vi "getFilePath.vi"(11 "fileName":string="VI\\SYSKON P4500 Init Config.vi") -> (3 "path":path=path "C:/Users/chen106/Desktop/vTestStudioCfgEditor/VI/SYSKON P4500 Init Config.vi")   [LabVIEW 2010]
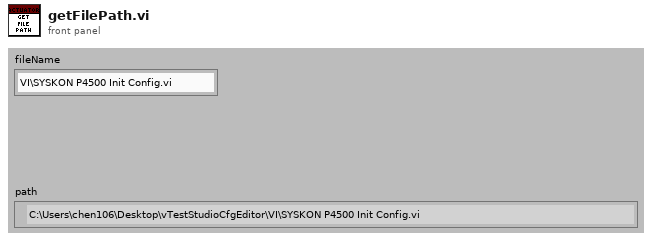
[diagram p1: front panel]
types:
  T1 = enum32{"invalid app kind", "Development System", "Run Time System", "Student Edition", "Embedded LabVIEW", "Evaluation", "Custom"}
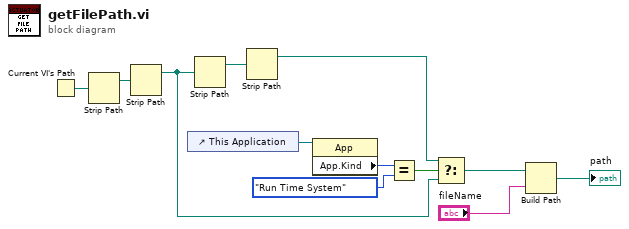
[diagram p0: block diagram]
diagram:
  n1 = Current VI's Path() -> (path=w12:path)
  n2 = Strip Path(path=w12) -> (stripped path=w10:path)  [unwired: 1 out]
  n3 = Strip Path(path=w10) -> (stripped path=w3:path)  [unwired: 1 out]
  n4 = control-ref of="This Application"() -> (w9:refnum<vi>)
  n5 = Strip Path(path=w3) -> (stripped path=w5:path)  [unwired: 1 out]
  n6 = Strip Path(path=w5) -> (stripped path=w4:path)  [unwired: 1 out]
  n7 = property class="App"(reference=w9) -> ("App.Kind"=w8:T1)  [unwired: 1 in, 2 out]
  n8 = Equal?(x=w8, y=T1."Run Time System" ("Application:Kind")) -> (x = y?=w6:bool)
  n9 = Select(t=w4, s=w6, f=w3) -> (s? t:f=w2:path)
  n10 = Build Path(base path=w2, name or relative path="fileName") -> (appended path=→"path":path)
